vi "Configure Shared LO Frequencies (Multi).vi"(0 "niUsrpRio Sessions":T2[](array[typedef]) {"Daughterboard Clock Rate" format="%#.3pHz"; "FPGA Data Clock Rate" format="%#.3pHz"; "Data Clock Rate" format="%#.3pHz"; "Characterization Data"."Frequencies [Hz]" format="%#_6p"; "EEPROM Characterization Header"."Pointer to Device Data Header" format="%x"; "EEPROM Characterization Header"."Checksum" format="%x"; "Device Data Header"."Pointer to Characterization Data" format="%x"; "Device Data Header"."Checksum" format="%x"; "EEPROM Header"."Pointer to User Header" format="%x"; "EEPROM Header"."Pointer to Factory Header" format="%x"; "EEPROM Header"."Product Code" format="%x"; "EEPROM Header"."Checksum" format="%x"}, 5 "coerced configs":T1(array[cluster]), 7 "rx configs":T12(array[cluster]), 11 "error in":errorcluster) -> (4 "niUsrpRio Sessions (out)":T2[](array[typedef]) {"Daughterboard Clock Rate" format="%#.3pHz"; "FPGA Data Clock Rate" format="%#.3pHz"; "Data Clock Rate" format="%#.3pHz"; "Characterization Data"."Frequencies [Hz]" format="%#_6p"; "EEPROM Characterization Header"."Pointer to Device Data Header" format="%x"; "EEPROM Characterization Header"."Checksum" format="%x"; "Device Data Header"."Pointer to Characterization Data" format="%x"; "Device Data Header"."Checksum" format="%x"; "EEPROM Header"."Pointer to User Header" format="%x"; "EEPROM Header"."Pointer to Factory Header" format="%x"; "EEPROM Header"."Product Code" format="%x"; "EEPROM Header"."Checksum" format="%x"}, 6 "coerced configs out":T1(array[cluster]), 15 "error out":errorcluster)   [LabVIEW 2020]
uses:
  Start Trigger.ctl
  <instrlib>/niUsrpRio/Config/v1/Host/Public/niUsrpRio Session.ctl
  <instrlib>/_niInstr/Register Bus/v0/Host/Public/Register Bus Session.ctl
  <instrlib>/_niInstr/Register Bus/v0/Host/Private/Session Data.ctl
  <instrlib>/niUsrpRio/Config/v1/Host/Private/DB Queue Reference.ctl
  <instrlib>/niUsrpRio/Config/v1/Host/Private/Daughterboard Data.ctl
  <instrlib>/niUsrpRio/Config/v1/Host/Private/ATR state data.ctl
  <instrlib>/niUsrpRio/Config/v1/Host/Private/Antenna Configuration.ctl
  <instrlib>/niUsrpRio/Config/v1/Host/Private/CPLD Power Mode.ctl
  <instrlib>/niUsrpRio/Config/v1/Host/Public/EEPROM Header.ctl
  <instrlib>/niUsrpRio/Config/v1/Host/Public/EEPROM Device Data Header.ctl
  <instrlib>/niUsrpRio/Config/v1/Host/Public/EEPROM Characterization Header.ctl
  <instrlib>/niUsrpRio/Config/v1/Host/Public/Characterization Data.ctl
  <instrlib>/niUsrpRio/Config/v1/Host/Public/IQ Imbalance.ctl
  <instrlib>/niUsrpRio/Config/v1/Host/Private/TwinRX LO.ctl
  <instrlib>/niUsrpRio/Config/v1/Host/niUsrpRio Config v1 Host.lvlib
  <instrlib>/niUsrpRio/Config/v1/Host/Private/niusrpriolv.lvlib
  <instrlib>/_niInstr/Register Bus/v0/Host/niInstr Register Bus v0 Host.lvlib
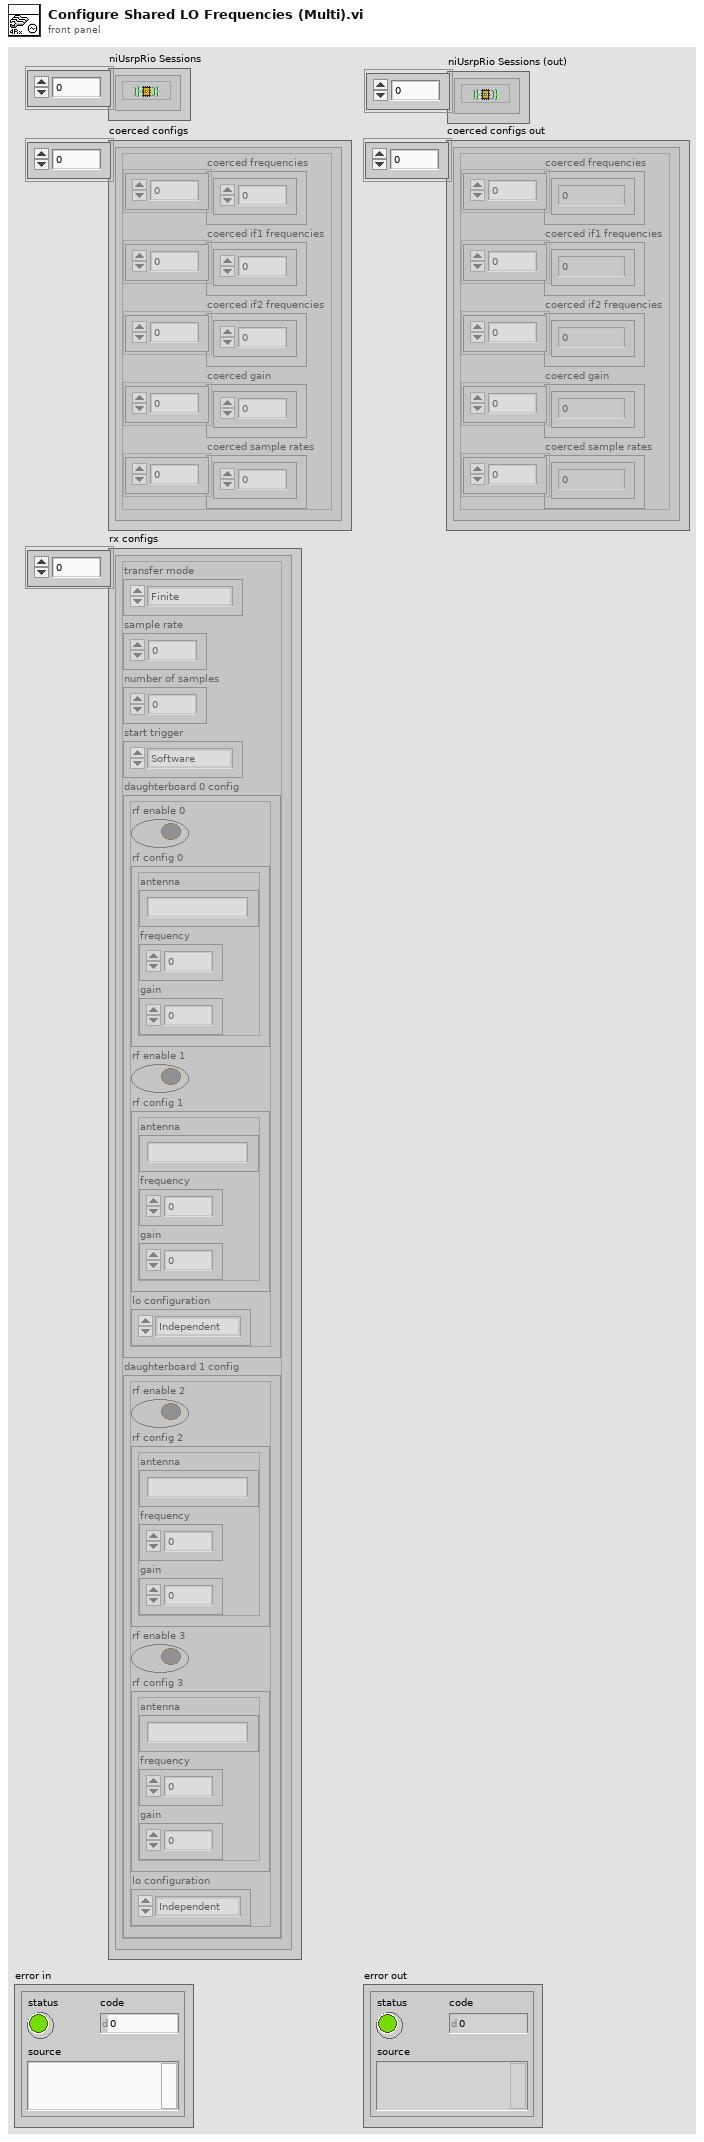
[diagram p1: front panel]
types:
  T1 = cluster{"coerced frequencies":dbl[], "coerced if1 frequencies":dbl[], "coerced if2 frequencies":dbl[], "coerced gain":dbl[], "coerced sample rates":dbl[]}[]
  T2 = typedef "niUsrpRio Config v1 Host.lvlib/niUsrpRio Session.ctl" = cluster{"FPGA Interface":refnum<k20>, "RIO Interface Number":u32, "Data Clock Rate":u32, "FPGA Data Clock Rate":u32, "Global Settings Register Bus":T3, "Radio 0 Settings Register Bus":T3, "Radio 1 Settings Register Bus":T3, "Radio Settings Bus Semaphore":T4, "DB Queues":T5[], "Characterization Data Valid?":bool, "EEPROM Header":T6, "Device Data Header":T7, "EEPROM Characterization Header":T8, "Characterization Data":T9[], "FPGA Current Version":u32, "FPGA Oldest Compatible Version":u32, "Fixed Logic Current Version":u32, "Fixed Logic Oldest Compatible Version":u32, "FPGA Radio Settings Bus Current Version":u32, "FPGA Radio Settings Bus Oldest Compatible Version":u32, "FPGA Board Config Current Version":u32, "FPGA Board Config Oldest Compatible Version":u32, "Daughterboard Clock Rate":u32, "daughterboard configuration session handles":u64[]}
  T3 = typedef "niInstr Register Bus v0 Host.lvlib/Register Bus Session.ctl" = refnum<queue>
  T4 = typedef "Semaphore RefNum" = refnum<k1>
  T5 = typedef "niUsrpRio Config v1 Host.lvlib/DB Queue Reference.ctl" = refnum<queue>
  T6 = typedef "niUsrpRio Config v1 Host.lvlib/EEPROM Header.ctl" = cluster{"Checksum":u32, "Product Code":u16, "Hardware Current Version":u16, "Hardware Oldest Compatible Version":u16, "EEPROM Map Current Version":u16, "EEPROM Map Oldest Compatible Version":u16, "User Password":string, "Pointer to Factory Header":u32, "Pointer to User Header":u32, "Recommended Interval":u16, "Number of Reserved Bytes":i32, "Number of Daughterboards":u8, "Daughterboard IDs":u16[], "Daughterboard Serial Numbers":string[]}
  T7 = typedef "niUsrpRio Config v1 Host.lvlib/EEPROM Device Data Header.ctl" = cluster{"Checksum":u32, "Number of Channels":u8, "Number of Gain Settings":u16[], "Pointer to Characterization Data":u32[], "Number of Reserved Bytes":i32, "Number of Frequencies":u16[]}
  T8 = typedef "niUsrpRio Config v1 Host.lvlib/EEPROM Characterization Header.ctl" = cluster{"Checksum":u32, "Date":timestamp, "Temperature":sgl, "Misc. Info":string, "Pointer to Device Data Header":u32, "Number of Reserved Bytes":i32}
  T9 = typedef "niUsrpRio Config v1 Host.lvlib/Characterization Data.ctl" = cluster{"Gains[dB]":dbl[], "Frequencies [Hz]":dbl[], "IQ Imbalance Table":T10[], "Measured Gains[dB]":dbl[][]}
  T10 = typedef "niUsrpRio Config v1 Host.lvlib/IQ Imbalance.ctl" = cluster{"Gain Imbalance [linear]":dbl, "Phase Imbalance [radians]":dbl, "Offset":cdb}
  T11 = typedef "Start Trigger.ctl" = enum8{"Software", "Digital Edge", "Rx Start Trigger", "Tx Start Trigger", "Immediate", "Future Time Event"}
  T12 = cluster{"transfer mode":enum16{"Finite", "Continuous"}, "sample rate":dbl, "number of samples":u32, "start trigger":T11, "daughterboard 0 config":cluster{"rf enable 0":bool, "rf config 0":cluster{"antenna":string, "frequency":dbl, "gain":dbl}, "rf enable 1":bool, "rf config 1":cluster{"antenna":string, "frequency":dbl, "gain":dbl}, "lo configuration":enum16{"Independent", "Import", "Shared and Export", "Reimport", "Shared"}}, "daughterboard 1 config":cluster{"rf enable 2":bool, "rf config 2":cluster{"antenna":string, "frequency":dbl, "gain":dbl}, "rf enable 3":bool, "rf config 3":cluster{"antenna":string, "frequency":dbl, "gain":dbl}, "lo configuration":enum16{"Independent", "Import", "Shared and Export", "Reimport", "Shared"}}}[]
  T13 = typedef "niUsrpRio Config v1 Host.lvlib/TwinRX LO.ctl" = enum16{"IF1", "IF2"}
  T14 = enum16{"Independent", "Import", "Shared and Export", "Reimport", "Shared"}[]
  T15 = enum16{"Independent", "Import", "Shared and Export", "Reimport", "Shared"}
  T16 = cluster{"importing?":bool, "frequency":dbl, "coerced frequency":dbl, "coerced if1 frequency":dbl, "coerced if2 frequency":dbl, "scope":string}[][]
  T17 = cluster{"coerced frequencies":dbl[], "coerced if1 frequencies":dbl[], "coerced if2 frequencies":dbl[], "coerced gain":dbl[], "coerced sample rates":dbl[]}
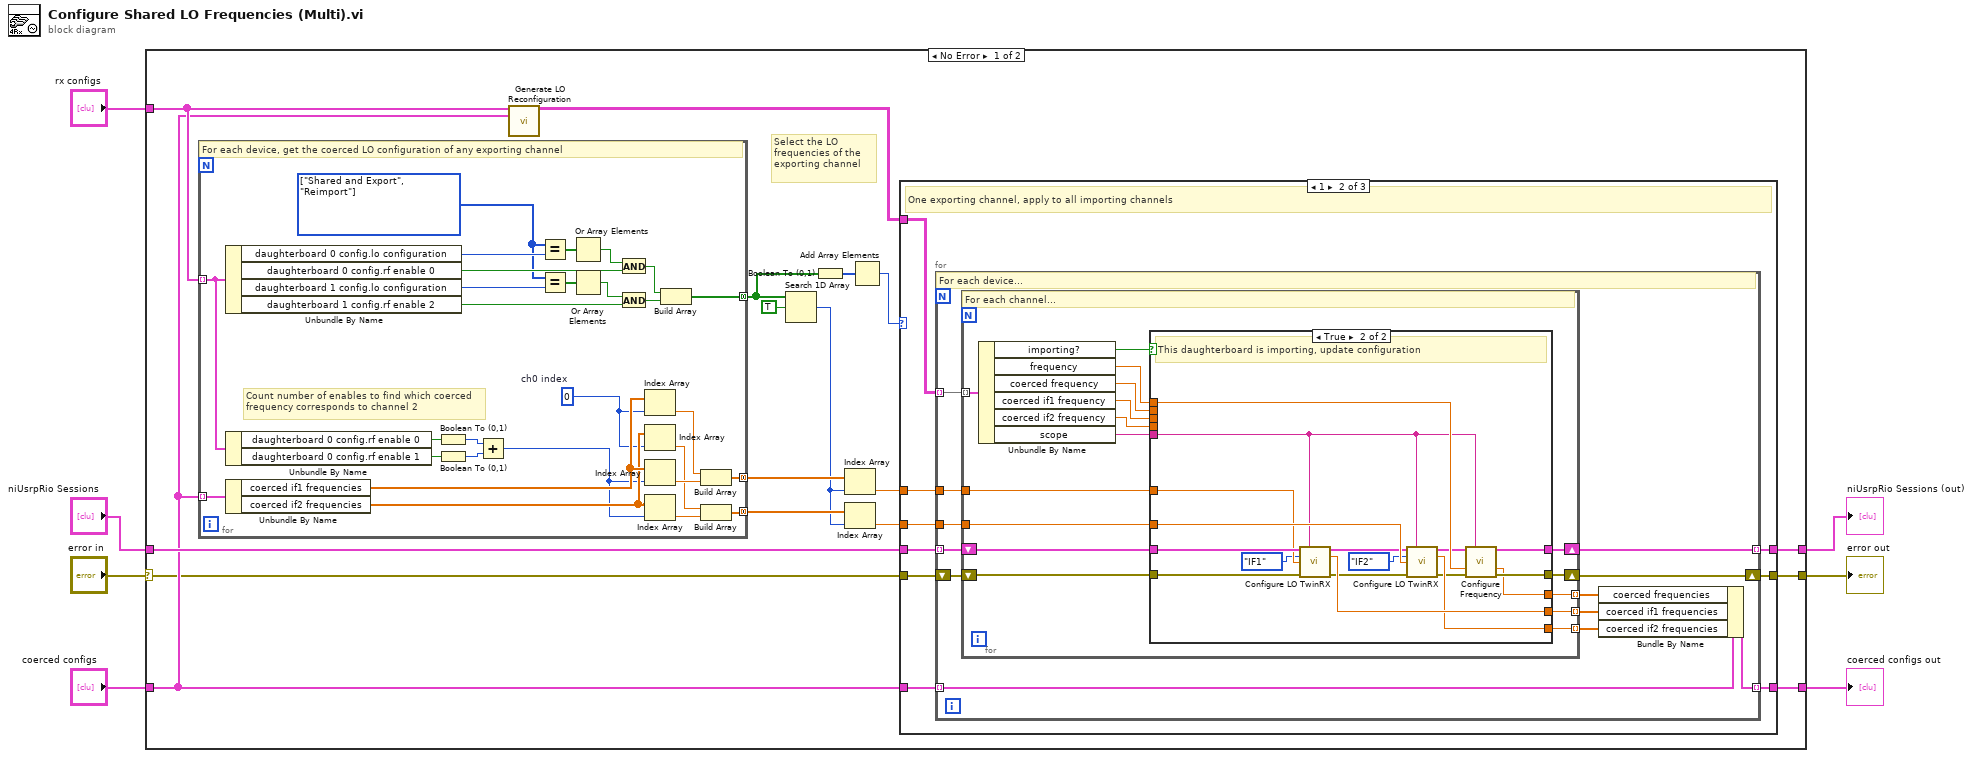
[diagram p0: block diagram]
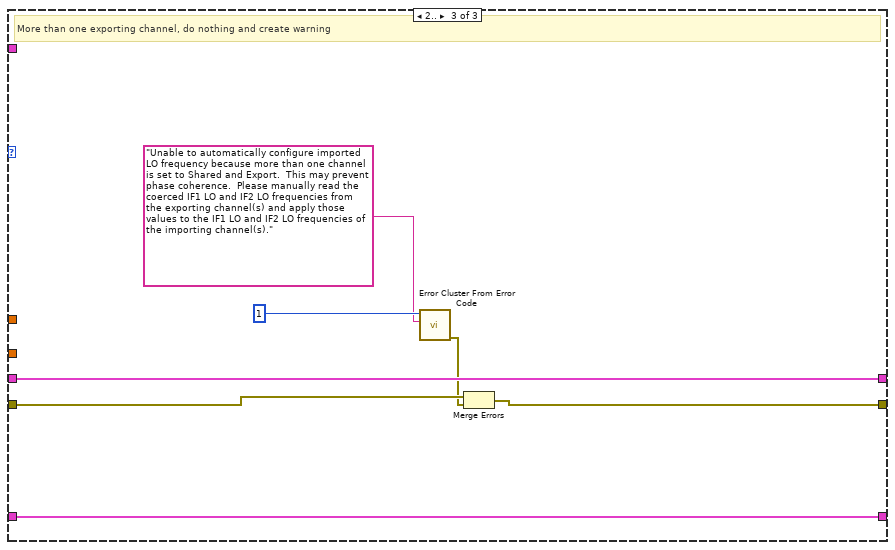
[diagram p4: hidden frame]
diagram:
  n1 = case shown="No Error" "error in" {
    selector: "error in" -> [w11 w124]
    tunnel: "niUsrpRio Sessions" -> [w18 w123]
    tunnel: [w17 w123] -> w6
    tunnel: [w16 w124] -> w5
    tunnel: "rx configs" -> [w15 _]
    tunnel: "coerced configs" -> [w13 w122]
    tunnel: [w12 w122] -> w2
    frame No Error {
      # "Select the LO frequencies of the exporting channel"
      n2 = for {
        tunnel: w15 -> [w47] mode=indexing
        tunnel: w13 -> [w46] mode=indexing
        tunnel: [w40] -> w23 mode=concatenating
        tunnel: [w42] -> w24 mode=concatenating
        tunnel: [w48] -> w9 mode=concatenating
        w26 = T14 [enum."Shared and Export", enum."Reimport"] items=["Independent", "Import", "Shared and Export", "Reimport", "Shared"]
        w37 = 0  # ch0 index
        # "Count number of enables to find which coerced frequency corresponds to channel 2"
        # "For each device, get the coerced LO configuration of any exporting channel"
        n3 = Unbundle By Name(w47) -> ("daughterboard 0 config.lo configuration"=w31:T15, "daughterboard 0 config.rf enable 0"=w52:bool, "daughterboard 1 config.lo configuration"=w25:T15, "daughterboard 1 config.rf enable 2"=w51:bool)
        n4 = Unbundle By Name(w47) -> ("daughterboard 0 config.rf enable 0"=w36:bool, "daughterboard 0 config.rf enable 1"=w35:bool)
        n5 = Unbundle By Name(w46) -> ("coerced if1 frequencies"=w45:dbl[], "coerced if2 frequencies"=w44:dbl[])
        n6 = Boolean To (0,1)(Boolean=w36) -> (0, 1=w34:i16)
        n7 = Boolean To (0,1)(Boolean=w35) -> (0, 1=w33:i16)
        n8 = Add(x=w34, y=w33) -> (x+y=w32:i16)
        n9 = Equal?(x=w26, y=w31) -> (x = y?=w30:bool[])
        n10 = Equal?(x=w26, y=w25) -> (x = y?=w28:bool[])
        n11 = Or Array Elements(Boolean array=w30) -> (logical OR=w29:bool)
        n12 = Or Array Elements(Boolean array=w28) -> (logical OR=w27:bool)
        n13 = And(x=w29, y=w52) -> (x .and. y?=w50:bool)
        n14 = And(x=w27, y=w51) -> (x .and. y?=w49:bool)
        n15 = Index Array(array=w45, index=w37) -> (element=w43:dbl)
        n16 = Index Array(array=w44, index=w37) -> (element=w39:dbl)
        n17 = Index Array(array=w45, index=w32) -> (element=w41:dbl)
        n18 = Index Array(array=w44, index=w32) -> (element=w38:dbl)
        n19 = Build Array(w50, w49) -> (w48:bool[])
        n20 = Build Array(w43, w41) -> (w42:dbl[])
        n21 = Build Array(w39, w38) -> (w40:dbl[])
      }
      n22 = call "Generate LO Reconfiguration.vi"("rx configs"=w15, "coerced configs"=w13) -> ("lo configs"=w14:T16)  [unwired: 13 in]
      n23 = Search 1D Array(1D array=w9, element=TRUE) -> (index of element=w22:i32)  [unwired: 1 in]
      n24 = Boolean To (0,1)(Boolean=w9) -> (0, 1=w10:i16[])
      n25 = Index Array(array=w24, index=w22) -> (element=w20:dbl)
      n26 = Index Array(array=w23, index=w22) -> (element=w19:dbl)
      n27 = Add Array Elements(numeric array=w10) -> (sum=w21:i16)
      n28 = case shown="1" w21 {
        tunnel: w20 -> [_ w62 _]
        tunnel: w19 -> [_ w63 _]
        tunnel: w11 -> [w54 w60 w120]
        tunnel: w18 -> [w55 w64 w121]
        tunnel: [w55 w61 w121] -> w17
        tunnel: [w54 w59 w119] -> w16
        tunnel: w14 -> [_ w58 _]
        tunnel: w13 -> [w53 w57 w115]
        tunnel: [w53 w56 w115] -> w12
        frame 0, Default {
          # "No exporting channel, do nothing"
        }
        frame 1 {
          # "One exporting channel, apply to all importing channels"
          n29 = for {
            tunnel: w64 -> [w74] mode=indexing
            tunnel: w63 -> [w72]
            tunnel: w62 -> [w73]
            tunnel: [w68] -> w61 mode=indexing
            shift-right: [w69] -> w59
            shift-left: w60 -> [w75]
            tunnel: w58 -> [w76] mode=indexing
            tunnel: w57 -> [w71] mode=indexing
            tunnel: [w70] -> w56 mode=indexing
            # "For each device..."
            n30 = for {
              tunnel: w72 -> [w91]
              tunnel: w73 -> [w90]
              shift-right: [w87] -> w68
              shift-left: w74 -> [w92]
              shift-right: [w88] -> w69
              shift-left: w75 -> [w89]
              tunnel: w76 -> [w86] mode=indexing
              tunnel: [w79] -> w67 mode=indexing
              tunnel: [w78] -> w66 mode=indexing
              tunnel: [w77] -> w65 mode=indexing
              # "For each channel..."
              n31 = Unbundle By Name(w86) -> ("importing?"=w85:bool, "frequency"=w84:dbl, "coerced frequency"=w82:dbl, "coerced if1 frequency"=w81:dbl, "coerced if2 frequency"=w80:dbl, "scope"=w83:string)
              n32 = case shown="True" w85 {
                tunnel: w92 -> [w96 w114]
                tunnel: w91 -> [_ w113]
                tunnel: w90 -> [_ w112]
                tunnel: w89 -> [w95 w111]
                tunnel: [w95 w110] -> w88
                tunnel: [w96 w109] -> w87
                tunnel: w84 -> [_ w108]
                tunnel: w82 -> [w97 _]
                tunnel: w83 -> [_ w107]
                tunnel: [w97 w106] -> w79
                tunnel: w81 -> [w94 _]
                tunnel: w80 -> [w93 _]
                tunnel: [w94 w105] -> w78
                tunnel: [w93 w104] -> w77
                frame False {
                  # "This daughterboard is not importing, keep old coerced values"
                }
                frame True {
                  # "This daughterboard is importing, update configuration"
                  n33 = call <instrlib>:"Configure LO TwinRX.vi"("niUsrpRio Session"=w114, "scope"=w107, "lo index"=TwinRX_LO."IF1", "frequency"=w112, "error in"=w111) -> ("niUsrpRio Session (out)"=w102:T2, "coerced frequency"=w105:dbl, "error out"=w103:errorcluster)  [unwired: 8 in]
                  n34 = call <instrlib>:"Configure LO TwinRX.vi"("niUsrpRio Session"=w102, "scope"=w107, "lo index"=TwinRX_LO."IF2", "frequency"=w113, "error in"=w103) -> ("niUsrpRio Session (out)"=w99:T2, "coerced frequency"=w104:dbl, "error out"=w98:errorcluster)  [unwired: 8 in]
                  n35 = call "Configure Frequency.vi"("niUsrpRio Session"=w99, "scope"=w107, "frequency"=w108, "error in"=w98) -> ("niUsrpRio Session (out)"=w109:T2, "coerced frequency"=w106:dbl, "error out"=w110:errorcluster)  [unwired: 8 in, 1 out]
                }
              }
            }
            n36 = Bundle By Name(cluster=w71, "coerced frequencies"=w67, "coerced if1 frequencies"=w66, "coerced if2 frequencies"=w65) -> (w70:T17)
          }
        }
        frame 2.. {
          # "More than one exporting channel, do nothing and create warning"
          n37 = call <vilib>:"Error Cluster From Error Code.vi"("error message (\"\")"="Unable to automatically configure imported LO frequency because more than one channel is set to Shared and Export.  This may prevent phase coherence.  Please manually read the coerced IF1 LO and IF2 LO frequencies from the exporting channel(s) and apply those values to the IF1 LO and IF2 LO frequencies of the importing channel(s)." ("error message (\"\")"), "error code (0)"=1) -> ("error out"=w118:errorcluster)  [unwired: 7 in]
          n38 = Merge Errors(w120, w118) -> (w119:errorcluster)
        }
      }
    }
    frame Error {
    }
  }
  "error out" <- w5
  "niUsrpRio Sessions (out)" <- w6
  "coerced configs out" <- w2
